vi "Get Active Pin Map Path.vi"(8 "error in (no error)":errorcluster, 11 "Session in":refnum<class "Plugin Session.lvclass">) -> (0 "error out":errorcluster, 2 "Active Pin Map Path":path, 3 "Session out":refnum<class "Plugin Session.lvclass">)   [LabVIEW 2020, in "InstrumentStudio Plugin SDK.lvlib" / "Plugin Session.lvclass"]
doc: "Call this VI to read the active pin map path in InstrumentStudio. If the active pin map does not exist or is \ninvalid, an empty path will be returned."
uses:
  Plugin Session.lvclass
  Plugin Session.lvclass/Plugin Session.ctl
  Read Session Id.vi
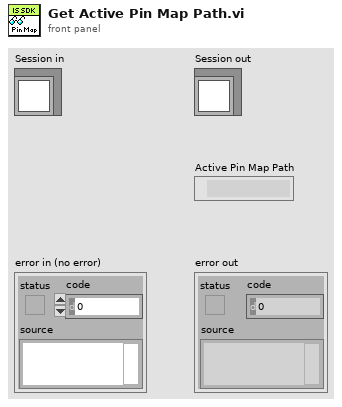
[diagram p1: front panel]
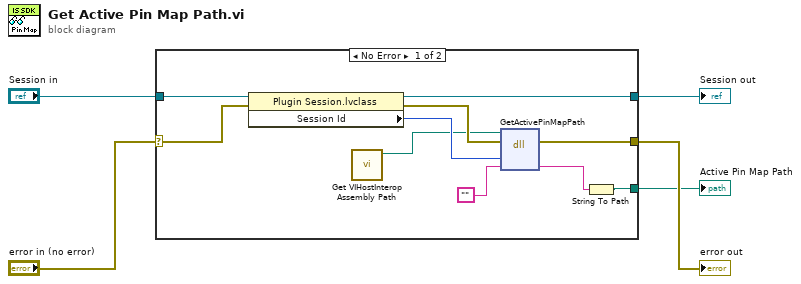
[diagram p0: block diagram]
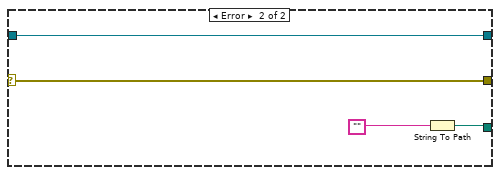
[diagram p2: hidden frame]
diagram:
  n1 = case shown="No Error" "error in (no error)" {
    selector: "error in (no error)" -> [w13 w18]
    tunnel: "Session in" -> [w15 w19]
    tunnel: [w14 w19] -> w2
    tunnel: [w10 w18] -> w4
    tunnel: [w7 w17] -> w1
    frame No Error {
      n2 = property class="Plugin Session.lvclass"(reference=w15, error in=w13) -> (reference out=w14:refnum<class "Plugin Session.lvclass">, error out=w12:errorcluster, "Session Id"=w11:u64)
      n3 = call "Get VIHostInterop Assembly Path.vi"() -> ("VIHost.Interop Assembly"=w8:path)  [unwired: 11 in]
      n4 = dll-call lib="C:/Dev/ASW/Source/InstrumentStudio/IFDistribution/VIHostPanel/objects/export/targets/win64U/x64/msvc-14.0/debug/NationalInstruments.VIHost.Interop.dll" fn="GetActivePinMapPath"(path in=w8, error in=w12, "sessionId"=w11, "pinMapPath"="") -> (error out=w10:errorcluster, "pinMapPath"=w6:string)  [unwired: 3 in, 1 out]
      n5 = String To Path(string=w6) -> (path=w7:path)
    }
    frame Error {
      n6 = String To Path(string="") -> (path=w17:path)
    }
  }
  "error out" <- w4
  "Session out" <- w2
  "Active Pin Map Path" <- w1
